vi "Text Detection Model (EAST).vi"(1 "Model Path Directory (Default: Relative to This VI)":path=path "") -> (0 "Text Detection Model (EAST)":T1)   [LabVIEW 2020]
uses:
  feature_detection/Text Detector/Model.ctl
  common/Image Size (Integer).ctl
  common/Object Point (Float).ctl
  common/common.lvlib
  feature_detection/Text Detector/Text Detector.lvclass
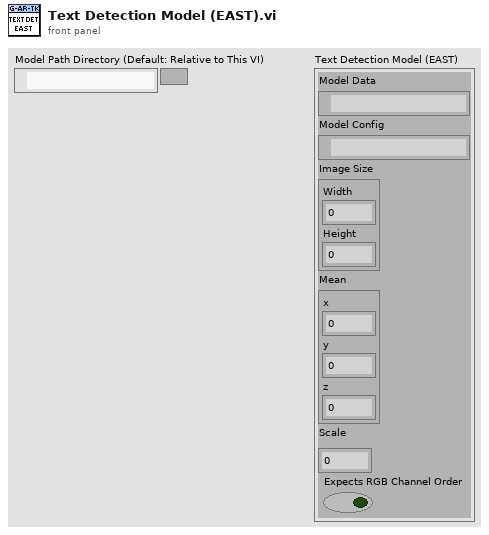
[diagram p1: front panel]
types:
  T1 = typedef "feature_detection.lvlib/Text Detector.lvclass/Model.ctl" = cluster{"Model Data":path, "Model Config":path, "Image Size":T2, "Mean":T3, "Scale":dbl, "Expects RGB Channel Order":bool}
  T2 = typedef "common.lvlib/Image Size (Integer).ctl" = cluster{"Width":u16, "Height":u16}
  T3 = typedef "common.lvlib/Object Point (Float).ctl" = cluster{"x":dbl, "y":dbl, "z":dbl}
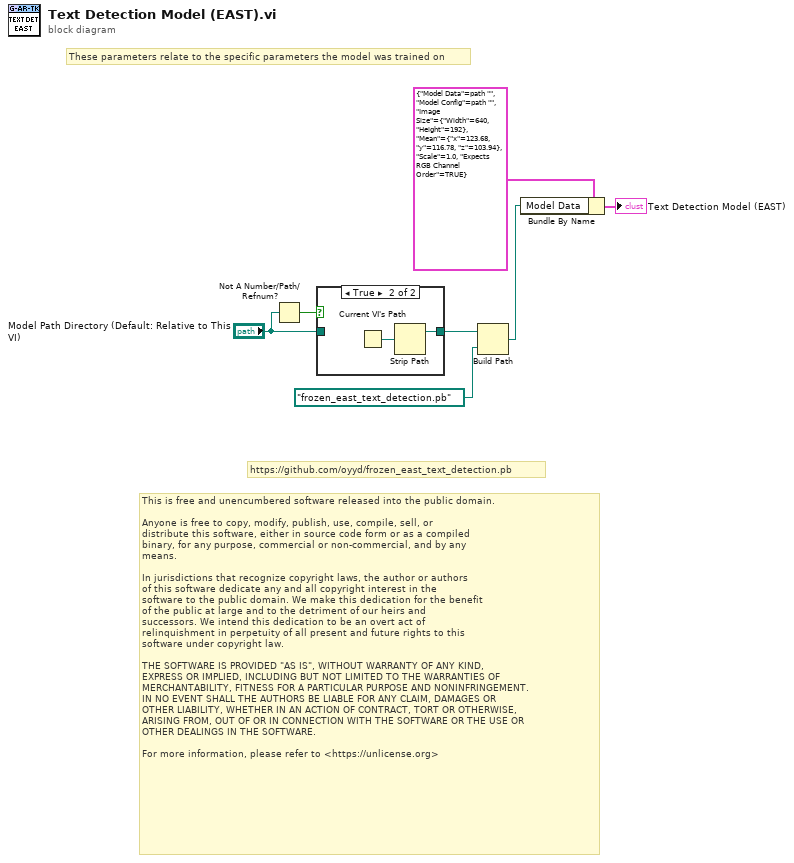
[diagram p0: block diagram]
diagram:
  # "This is free and unencumbered software released into the public domain.\n\nAnyone is free to copy, modify, publish, use, compile, sell, or\ndistribute this software, either in source code form or as a compiled\nbinary, for any purpose, commercial or non-commercial, and by any\nmeans.\n\nIn jurisdictions that recognize copyright laws, the author or authors\nof this software dedicate any and all copyright interest in the\nsoftware to the public domain. We make this dedication for the benefit\nof the public at large and to the detriment of our heirs and\nsuccessors. We intend this dedication to be an overt act of\nrelinquishment in perpetuity of all present and future rights to this\nsoftware under copyright law.\n\nTHE SOFTWARE IS PROVIDED \"AS IS\", WITHOUT WARRANTY OF ANY KIND,\nEXPRESS OR IMPLIED, INCLUDING BUT NOT LIMITED TO THE WARRANTIES OF\nMERCHANTABILITY, FITNESS FOR A PARTICULAR PURPOSE AND NONINFRINGEMENT.\nIN NO EVENT SHALL THE AUTHORS BE LIABLE FOR ANY CLAIM, DAMAGES OR\nOTHER LIABILITY, WHETHER IN AN ACTION OF CONTRACT, TORT OR OTHERWISE,\nARISING FROM, OUT OF OR IN CONNECTION WITH THE SOFTWARE OR THE USE OR\nOTHER DEALINGS IN THE SOFTWARE.\n\nFor more information, please refer to <https://unlicense.org>"
  # "https://github.com/oyyd/frozen_east_text_detection.pb"
  # "These parameters relate to the specific parameters the model was trained on"
  n1 = Not A Number/Path/Refnum?(number/path/refnum="Model Path Directory (Default: Relative to This VI)") -> (NaN/Path/Refnum?=w5:bool)
  n2 = case shown="True" w5 {
    tunnel: [w8 w10] -> w4
    tunnel: "Model Path Directory (Default: Relative to This VI)" -> [w8 _]
    frame False {
    }
    frame True {
      n3 = Current VI's Path() -> (path=w9:path)
      n4 = Strip Path(path=w9) -> (stripped path=w10:path)  [unwired: 1 out]
    }
  }
  n5 = Build Path(base path=w4, name or relative path=path "frozen_east_text_detection.pb" ("Path")) -> (appended path=w1:path)
  n6 = Bundle By Name(cluster=T1 {"Model Data"=path "", "Model Config"=path "", "Image Size"={"Width"=640, "Height"=192}, "Mean"={"x"=123.68, "y"=116.78, "z"=103.94}, "Scale"=1.0, "Expects RGB Channel Order"=TRUE} ("output cluster"), "Model Data"=w1) -> (→"Text Detection Model (EAST)":T1)
